vi "Channel Mng Update Test Cases.vi"() -> (0 "error out":errorcluster, 2 "status":string, 3 "pass":bool)   [LabVIEW 2021]
uses:
  <vilib>/CIF Foundation/CIF Channels Core/CIF_NIChn/Double/CIF_NIChn_Double.lvclass
  C:/Program Files/National Instruments/LabVIEW 2021/vi.lib/CIF Foundation/CIF Channels Core/CIFChannels/CIFChannels.lvclass
  <vilib>/CIF Foundation/CIF Channels Core/CIFChannels/Typedef/Direction.ctl
  OOB/OOB_Rx/CIFCoreOOB_Rx.lvclass/CIFCoreOOB_Rx.ctl
  <vilib>/CIF Foundation/CIF Out of Band Commands/CIFOutOfBand.lvclass/CIFOutOfBand.ctl
  <vilib>/CIF Foundation/CIF Channels Core/CIFChannels/CIFChannels.lvclass
  <vilib>/CIF Foundation/CIF Channels Core/CIFChannels/CIFChannels.lvclass/CIFChannels.ctl
  Channels/CIFChannelMng/CIFChannelMng.lvclass/CIFChannelMng.ctl
  OOB/OOB_Rx/Private/Command Settings.vi
  <vilib>/CIF Foundation/CIF Out of Band Commands/Accessors/Write Local OOB Data.vi
  <vilib>/CIF Foundation/CIF Channels Core/ChannelCommon/Utilities/Add Error.vi
  <vilib>/CIF Foundation/CIF Channels Core/CIFChannels/Accessors/Read Name.vi
  <vilib>/CIF Foundation/CIF Channels Core/CIFChannels/Accessors/Read Custom Config Data.vi
  <vilib>/CIF Foundation/CIF Channels Core/CIFChannels/Accessors/Read Type.vi
  <vilib>/CIF Foundation/CIF Channels Core/CIFChannels/Accessors/Read Multi-Writer.vi
  <vilib>/CIF Foundation/CIF Channels Core/CIFChannels/Accessors/Read Direction.vi
  <vilib>/CIF Foundation/CIF Channels Core/CIFChannels/Accessors/Read Channel State.vi
  Channels/CIFChannelMng/Utilities/Get Channel Index by Name.vi
  Channels/CIFChannelMng/Utilities/Remove Channel by Index.vi
  <vilib>/CIF Foundation/CIF Channels Core/CIFChannels/Accessors/Read Tag Forced.vi
  <vilib>/CIF Foundation/CIF Utilities/Errors/Append Error Location.vi
  <vilib>/CIF Foundation/CIF Channels Core/CIFChannels/Accessors/Write Channel State.vi
  OOB/OOB_Rx/CIFCoreOOB_Rx.lvclass
  C:/Program Files/National Instruments/LabVIEW 2021/vi.lib/CIF Foundation/CIF Out of Band Commands/CIFOutOfBand.lvclass
  <vilib>/CIF Foundation/CIF Out of Band Commands/Init OOB.vi
  <vilib>/CIF Foundation/CIF Channels Core/CIFChannels/Core/Set Force.vi
  OOB/OOB_Rx/Typedef/FIFO Publisher.ctl
  <vilib>/CIF Foundation/CIF Channels Core/ChannelCommon/typedef/New FIFO Instance Configuration.ctl
  OOB/OOB_Rx/Typedef/Channel Connection Data.ctl
  Channels/CIFChannelMng/CIFChannelMng.lvclass
  <vilib>/CIF Foundation/CIF Channels Core/CIF_NIChn/FIFO_U8_Multi/CIF_Fifo_U8_Multi.lvclass
  <vilib>/CIF Foundation/CIF Channels Core/ChannelCommon/ChannelCommon.lvlib
  <vilib>/CIF Foundation/CIF Out of Band Commands/CIFOutOfBand.lvclass
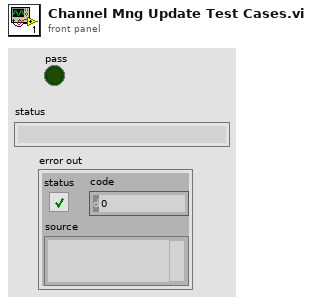
[diagram p1: front panel]
types:
  T1 = typedef "CIFChannels.lvclass/Direction.ctl" = enum16{"Publisher", "Subscriber"}
  T2 = typedef "CIFCoreOOB_Rx.lvclass/Channel Connection Data.ctl" = cluster{"Publisher Name":string, "Subscriber Name":string, "Connection Data":u8[]}
  T3 = typedef "CIFCoreOOB_Rx.lvclass/FIFO Publisher.ctl" = cluster{"Publisher Name":string, "New FIFO Instance Config":T4}
  T4 = typedef "ChannelCommon.lvlib/New FIFO Instance Configuration.ctl" = cluster{"Primary":bool, "Backpressure":bool, "Message/FIFO Override":u32}
  T5 = typedef "ChnMngOOB_Tx.lvclass/FIFO Publisher Return.ctl" = cluster{"FIFO Pub Name":string, "error":errorcluster, "Added":bool}
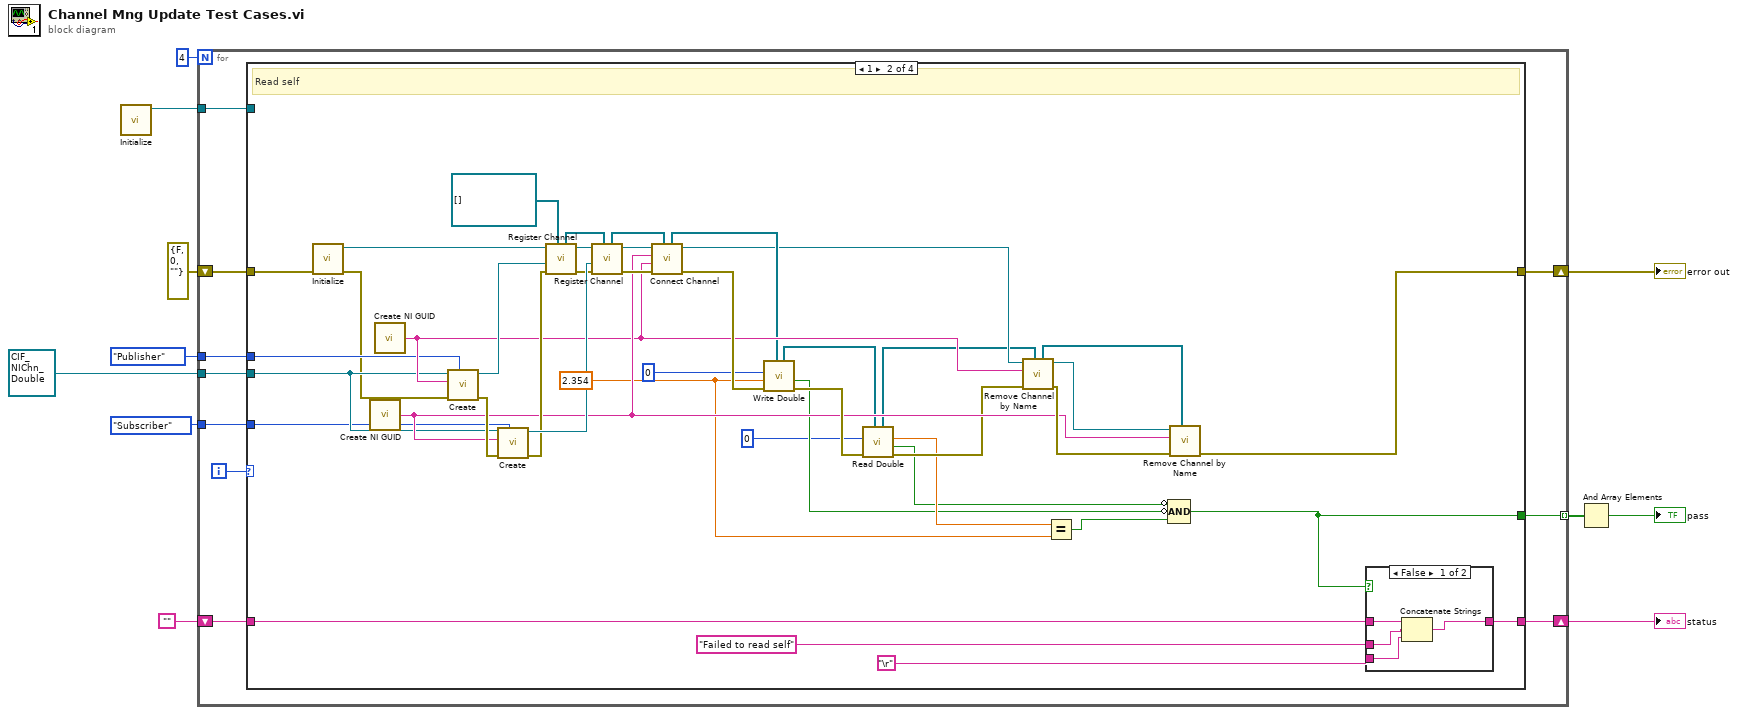
[diagram p0: block diagram]
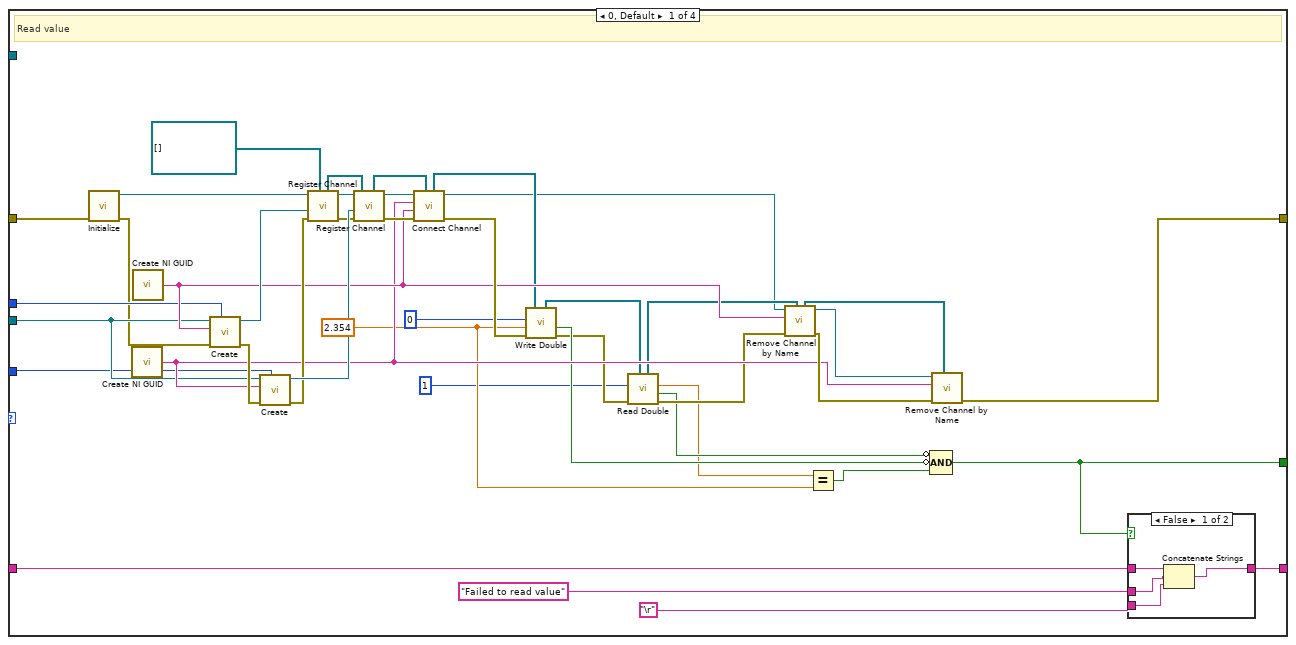
[diagram p2: hidden frame]
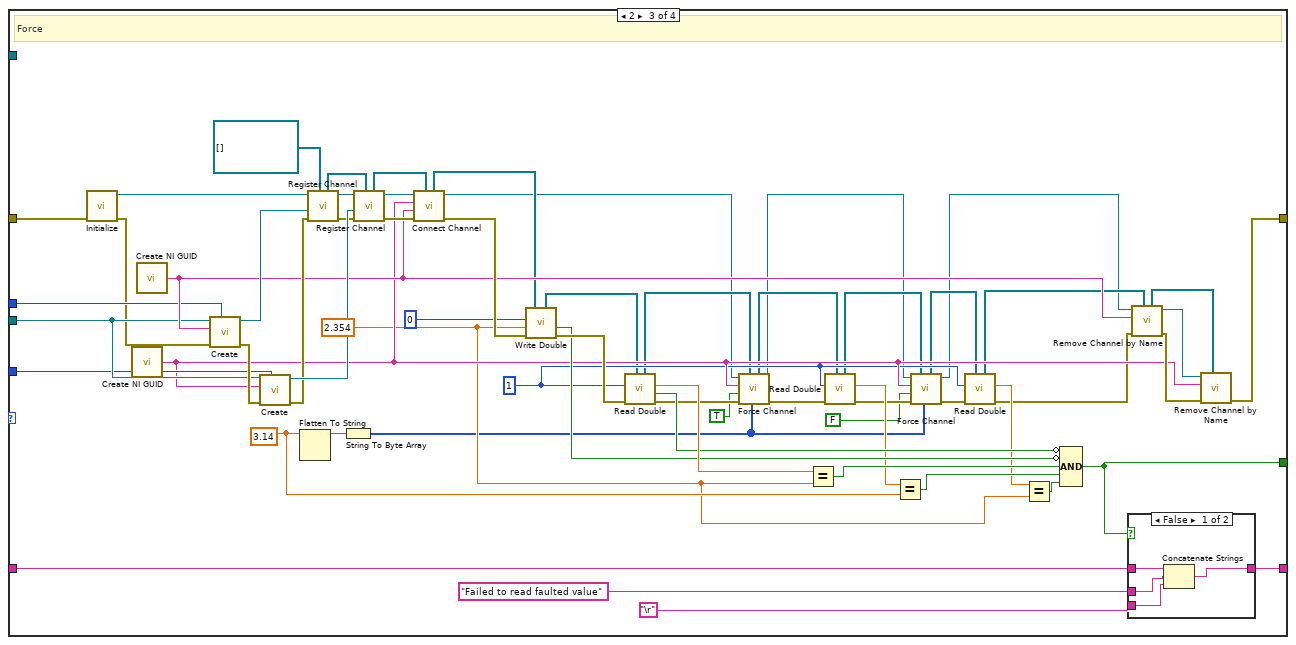
[diagram p5: hidden frame]
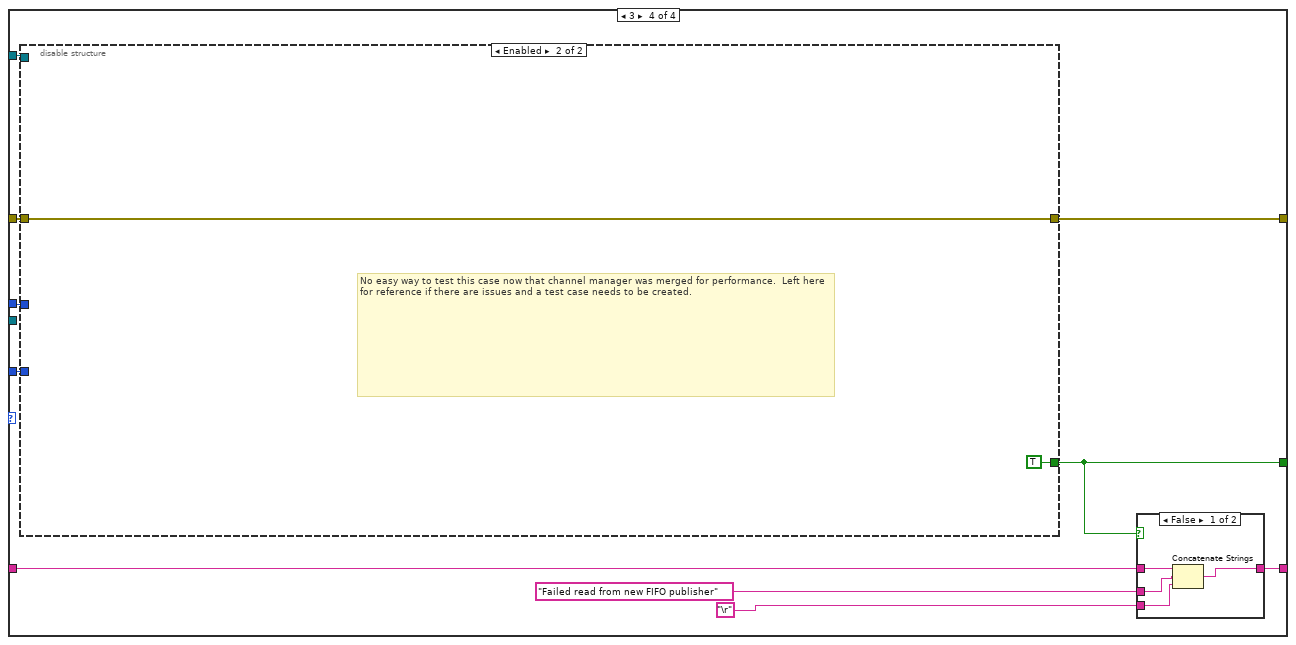
[diagram p7: hidden frame]
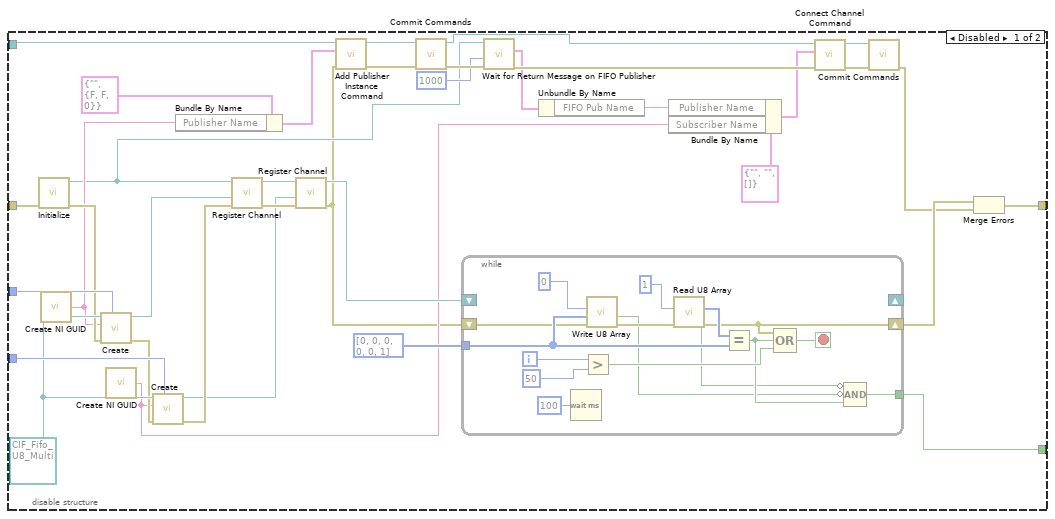
[diagram p8: hidden frame]
diagram:
  n1 = call "Initialize.vi"() -> ("CoreOOB_Rx out"=w1:refnum<class "CIFCoreOOB_Rx.lvclass">)  [unwired: 10 in, 1 out]
  n2 = for {
    N: 4 -> [_]
    tunnel: [w21] -> w11 mode=indexing
    shift-right: [w19] -> w6
    shift-left: errorcluster {"status"=FALSE, "code"=0, "source"=""} ("error out") -> [w20]
    shift-right: [w16] -> w7
    shift-left: "" -> [w17]
    tunnel: refnum<class "CIF_NIChn_Double.lvclass"> refnum ("CIF_NIChn_Double.lvclass") -> [w15]
    tunnel: Direction."Subscriber" ("Direction") -> [w14]
    tunnel: Direction."Publisher" ("Direction") -> [w13]
    tunnel: w1 -> [w12]
    i -> [w18]
    n3 = case shown="1" w18 {
      tunnel: [w58 w105 w171 w187] -> w21
      tunnel: w20 -> [w31 w79 w131 w189]
      tunnel: [w45 w92 w158 w183] -> w19
      tunnel: w17 -> [w63 w110 w176 w186]
      tunnel: [w62 w109 w175 w188] -> w16
      tunnel: w15 -> [w41 w84 w153 _]
      tunnel: w14 -> [w40 w83 w152 w190]
      tunnel: w13 -> [w39 w82 w151 w191]
      tunnel: w12 -> [_ _ _ w182]
      frame 0, Default {
        w43 = 2.354
        # "Read value"
        n4 = call "Initialize.vi"("error in (no error)"=w31) -> ("error out"=w30:errorcluster, "CIFChannelMng out"=w32:refnum<class "CIFChannelMng.lvclass">)  [unwired: 9 in]
        n5 = call <vilib>:"Create NI GUID.vi"() -> ("NI GUID"=w44:string)
        n6 = call <vilib>:"Create NI GUID.vi"() -> ("NI GUID"=w48:string)
        n7 = call-dynamic "Create.vi"("Direction"=w39, "error in (no error)"=w30, "Name"=w48, "CIFTag in"=w41) -> ("error out"=w53:errorcluster, "CIFTag out"=w52:refnum<class "CIF_NIChn_Double.lvclass">)  [unwired: 6 in]
        n8 = call-dynamic "Create.vi"("Direction"=w40, "error in (no error)"=w53, "Name"=w44, "CIFTag in"=w41) -> ("error out"=w54:errorcluster, "CIFTag out"=w57:refnum<class "CIF_NIChn_Double.lvclass">)  [unwired: 6 in]
        n9 = call "Register Channel.vi"("Channel Array in"=refnum<class "CIFChannels.lvclass">[] [], "error in (no error)"=w54, "Channel"=w52, "CIFChannelMng in"=w32) -> ("error out"=w51:errorcluster, "CIFChannelMng out"=w50:refnum<class "CIFChannelMng.lvclass">, "Channel Array out"=w23:refnum<class "CIFChannels.lvclass">[])  [unwired: 4 in, 1 out]
        n10 = call "Register Channel.vi"("Channel Array in"=w23, "error in (no error)"=w51, "Channel"=w57, "CIFChannelMng in"=w50) -> ("error out"=w56:errorcluster, "CIFChannelMng out"=w55:refnum<class "CIFChannelMng.lvclass">, "Channel Array out"=w22:refnum<class "CIFChannels.lvclass">[])  [unwired: 4 in, 1 out]
        n11 = call "Connect Channel.vi"("Channel Array in"=w22, "error in (no error)"=w56, "Publisher Name"=w48, "Subscriber Name"=w44, "CIFChannelMng in"=w55) -> ("error out"=w49:errorcluster, "CIFChannelMng out"=w26:refnum<class "CIFChannelMng.lvclass">, "Channel Array out"=w29:refnum<class "CIFChannels.lvclass">[])  [unwired: 3 in, 1 out]
        n12 = call "Write Double.vi"("Channel Array in"=w29, "error in (no error)"=w49, "Data"=w43, "Channel Index"=0) -> ("error out"=w37:errorcluster, "timed out?"=w42:bool, "Channel Array out"=w28:refnum<class "CIFChannels.lvclass">[])  [unwired: 5 in]
        n13 = call "Read Double.vi"("Channel Array in"=w28, "error in (no error)"=w37, "Channel Index"=1 ("Index")) -> ("error out"=w38:errorcluster, "timed out?"=w35:bool, "Data"=w34:dbl, "Channel Array out"=w27:refnum<class "CIFChannels.lvclass">[])  [unwired: 5 in]
        n14 = call "Remove Channel by Name.vi"("Channel Array in"=w27, "error in (no error)"=w38, "Channel Name"=w48, "CIFChannelMng in"=w26) -> ("error out"=w47:errorcluster, "CIFChannelMng out"=w46:refnum<class "CIFChannelMng.lvclass">, "Channel Array out"=w25:refnum<class "CIFChannels.lvclass">[])  [unwired: 4 in, 1 out]
        n15 = Equal?(x=w34, y=w43) -> (x = y?=w59:bool)
        n16 = Compound Arithmetic op=AND(invert w35, invert w42, w59) -> (w58:bool)
        n17 = call "Remove Channel by Name.vi"("Channel Array in"=w25, "error in (no error)"=w47, "Channel Name"=w44, "CIFChannelMng in"=w46) -> ("error out"=w45:errorcluster)  [unwired: 4 in, 3 out]
        n18 = case shown="False" w58 {
          tunnel: w63 -> [w67 w68]
          tunnel: [w64 w68] -> w62
          tunnel: "Failed to read value" -> [w66 _]
          tunnel: "\r" -> [w65 _]
          frame False {
            n19 = Concatenate Strings(w67, w66, w65) -> (w64:string)
          }
          frame True {
          }
        }
      }
      frame 1 {
        w88 = 2.354
        # "Read self"
        n20 = call "Initialize.vi"("error in (no error)"=w79) -> ("error out"=w77:errorcluster, "CIFChannelMng out"=w78:refnum<class "CIFChannelMng.lvclass">)  [unwired: 9 in]
        n21 = call <vilib>:"Create NI GUID.vi"() -> ("NI GUID"=w91:string)
        n22 = call <vilib>:"Create NI GUID.vi"() -> ("NI GUID"=w85:string)
        n23 = call-dynamic "Create.vi"("Direction"=w82, "error in (no error)"=w77, "Name"=w85, "CIFTag in"=w84) -> ("error out"=w100:errorcluster, "CIFTag out"=w99:refnum<class "CIF_NIChn_Double.lvclass">)  [unwired: 6 in]
        n24 = call-dynamic "Create.vi"("Direction"=w83, "error in (no error)"=w100, "Name"=w91, "CIFTag in"=w84) -> ("error out"=w101:errorcluster, "CIFTag out"=w104:refnum<class "CIF_NIChn_Double.lvclass">)  [unwired: 6 in]
        n25 = call "Register Channel.vi"("Channel Array in"=refnum<class "CIFChannels.lvclass">[] [], "error in (no error)"=w101, "Channel"=w99, "CIFChannelMng in"=w78) -> ("error out"=w98:errorcluster, "CIFChannelMng out"=w97:refnum<class "CIFChannelMng.lvclass">, "Channel Array out"=w76:refnum<class "CIFChannels.lvclass">[])  [unwired: 4 in, 1 out]
        n26 = call "Register Channel.vi"("Channel Array in"=w76, "error in (no error)"=w98, "Channel"=w104, "CIFChannelMng in"=w97) -> ("error out"=w103:errorcluster, "CIFChannelMng out"=w102:refnum<class "CIFChannelMng.lvclass">, "Channel Array out"=w75:refnum<class "CIFChannels.lvclass">[])  [unwired: 4 in, 1 out]
        n27 = call "Connect Channel.vi"("Channel Array in"=w75, "error in (no error)"=w103, "Publisher Name"=w85, "Subscriber Name"=w91, "CIFChannelMng in"=w102) -> ("error out"=w96:errorcluster, "CIFChannelMng out"=w71:refnum<class "CIFChannelMng.lvclass">, "Channel Array out"=w73:refnum<class "CIFChannels.lvclass">[])  [unwired: 3 in, 1 out]
        n28 = call "Write Double.vi"("Channel Array in"=w73, "error in (no error)"=w96, "Data"=w88, "Channel Index"=0) -> ("error out"=w95:errorcluster, "timed out?"=w86:bool, "Channel Array out"=w70:refnum<class "CIFChannels.lvclass">[])  [unwired: 5 in]
        n29 = call "Read Double.vi"("Channel Array in"=w70, "error in (no error)"=w95, "Channel Index"=0) -> ("error out"=w90:errorcluster, "timed out?"=w87:bool, "Data"=w89:dbl, "Channel Array out"=w69:refnum<class "CIFChannels.lvclass">[])  [unwired: 5 in]
        n30 = call "Remove Channel by Name.vi"("Channel Array in"=w69, "error in (no error)"=w90, "Channel Name"=w85, "CIFChannelMng in"=w71) -> ("error out"=w94:errorcluster, "CIFChannelMng out"=w93:refnum<class "CIFChannelMng.lvclass">, "Channel Array out"=w72:refnum<class "CIFChannels.lvclass">[])  [unwired: 4 in, 1 out]
        n31 = Equal?(x=w89, y=w88) -> (x = y?=w106:bool)
        n32 = Compound Arithmetic op=AND(invert w87, invert w86, w106) -> (w105:bool)
        n33 = call "Remove Channel by Name.vi"("Channel Array in"=w72, "error in (no error)"=w94, "Channel Name"=w91, "CIFChannelMng in"=w93) -> ("error out"=w92:errorcluster)  [unwired: 4 in, 3 out]
        n34 = case shown="False" w105 {
          tunnel: w110 -> [w114 w115]
          tunnel: [w111 w115] -> w109
          tunnel: "Failed to read self" -> [w113 _]
          tunnel: "\r" -> [w112 _]
          frame False {
            n35 = Concatenate Strings(w114, w113, w112) -> (w111:string)
          }
          frame True {
          }
        }
      }
      frame 2 {
        w143 = 3.14
        w138 = 1 ("Channel Index")
        w135 = 2.354
        # "Force"
        n36 = call "Initialize.vi"("error in (no error)"=w131) -> ("error out"=w130:errorcluster, "CIFChannelMng out"=w132:refnum<class "CIFChannelMng.lvclass">)  [unwired: 9 in]
        n37 = call <vilib>:"Create NI GUID.vi"() -> ("NI GUID"=w140:string)
        n38 = call <vilib>:"Create NI GUID.vi"() -> ("NI GUID"=w154:string)
        n39 = call-dynamic "Create.vi"("Direction"=w151, "error in (no error)"=w130, "Name"=w154, "CIFTag in"=w153) -> ("error out"=w166:errorcluster, "CIFTag out"=w165:refnum<class "CIF_NIChn_Double.lvclass">)  [unwired: 6 in]
        n40 = call-dynamic "Create.vi"("Direction"=w152, "error in (no error)"=w166, "Name"=w140, "CIFTag in"=w153) -> ("error out"=w167:errorcluster, "CIFTag out"=w170:refnum<class "CIF_NIChn_Double.lvclass">)  [unwired: 6 in]
        n41 = Flatten To String(anything=w143) -> (data string=w147:string)  [unwired: 3 in, 2 out]
        n42 = call "Register Channel.vi"("Channel Array in"=refnum<class "CIFChannels.lvclass">[] [], "error in (no error)"=w167, "Channel"=w165, "CIFChannelMng in"=w132) -> ("error out"=w164:errorcluster, "CIFChannelMng out"=w163:refnum<class "CIFChannelMng.lvclass">, "Channel Array out"=w128:refnum<class "CIFChannels.lvclass">[])  [unwired: 4 in, 1 out]
        n43 = String To Byte Array(string=w147) -> (unsigned byte array=w133:u8[])
        n44 = call "Register Channel.vi"("Channel Array in"=w128, "error in (no error)"=w164, "Channel"=w170, "CIFChannelMng in"=w163) -> ("error out"=w169:errorcluster, "CIFChannelMng out"=w168:refnum<class "CIFChannelMng.lvclass">, "Channel Array out"=w127:refnum<class "CIFChannels.lvclass">[])  [unwired: 4 in, 1 out]
        n45 = call "Connect Channel.vi"("Channel Array in"=w127, "error in (no error)"=w169, "Publisher Name"=w154, "Subscriber Name"=w140, "CIFChannelMng in"=w168) -> ("error out"=w162:errorcluster, "CIFChannelMng out"=w118:refnum<class "CIFChannelMng.lvclass">, "Channel Array out"=w126:refnum<class "CIFChannels.lvclass">[])  [unwired: 3 in, 1 out]
        n46 = call "Write Double.vi"("Channel Array in"=w126, "error in (no error)"=w162, "Data"=w135, "Channel Index"=0) -> ("error out"=w161:errorcluster, "timed out?"=w155:bool, "Channel Array out"=w125:refnum<class "CIFChannels.lvclass">[])  [unwired: 5 in]
        n47 = call "Read Double.vi"("Channel Array in"=w125, "error in (no error)"=w161, "Channel Index"=w138) -> ("error out"=w149:errorcluster, "timed out?"=w156:bool, "Data"=w157:dbl, "Channel Array out"=w124:refnum<class "CIFChannels.lvclass">[])  [unwired: 5 in]
        n48 = call "Force Channel.vi"("Force Data"=w133, "Channel Array in"=w124, "error in (no error)"=w149, "Force Active"=TRUE ("Fault Active"), "Channel Name"=w140, "CIFChannelMng in"=w118) -> ("error out"=w146:errorcluster, "CIFChannelMng out"=w117:refnum<class "CIFChannelMng.lvclass">, "Channel Array out"=w123:refnum<class "CIFChannels.lvclass">[])  [unwired: 2 in, 1 out]
        n49 = Equal?(x=w157, y=w135) -> (x = y?=w172:bool)
        n50 = call "Read Double.vi"("Channel Array in"=w123, "error in (no error)"=w146, "Channel Index"=w138) -> ("error out"=w142:errorcluster, "Data"=w144:dbl, "Channel Array out"=w122:refnum<class "CIFChannels.lvclass">[])  [unwired: 5 in, 1 out]
        n51 = Equal?(x=w144, y=w143) -> (x = y?=w145:bool)
        n52 = call "Force Channel.vi"("Force Data"=w133, "Channel Array in"=w122, "error in (no error)"=w142, "Force Active"=FALSE ("Fault Active"), "Channel Name"=w140, "CIFChannelMng in"=w117) -> ("error out"=w141:errorcluster, "CIFChannelMng out"=w116:refnum<class "CIFChannelMng.lvclass">, "Channel Array out"=w121:refnum<class "CIFChannels.lvclass">[])  [unwired: 2 in, 1 out]
        n53 = call "Read Double.vi"("Channel Array in"=w121, "error in (no error)"=w141, "Channel Index"=w138) -> ("error out"=w134:errorcluster, "Data"=w136:dbl, "Channel Array out"=w120:refnum<class "CIFChannels.lvclass">[])  [unwired: 5 in, 1 out]
        n54 = Equal?(x=w136, y=w135) -> (x = y?=w137:bool)
        n55 = Compound Arithmetic op=AND(invert w156, invert w155, w172, w145, w137) -> (w171:bool)
        n56 = case shown="False" w171 {
          tunnel: w176 -> [w180 w181]
          tunnel: [w177 w181] -> w175
          tunnel: "Failed to read faulted value" -> [w179 _]
          tunnel: "\r" -> [w178 _]
          frame False {
            n57 = Concatenate Strings(w180, w179, w178) -> (w177:string)
          }
          frame True {
          }
        }
        n58 = call "Remove Channel by Name.vi"("Channel Array in"=w120, "error in (no error)"=w134, "Channel Name"=w154, "CIFChannelMng in"=w116) -> ("error out"=w160:errorcluster, "CIFChannelMng out"=w159:refnum<class "CIFChannelMng.lvclass">, "Channel Array out"=w119:refnum<class "CIFChannels.lvclass">[])  [unwired: 4 in, 1 out]
        n59 = call "Remove Channel by Name.vi"("Channel Array in"=w119, "error in (no error)"=w160, "Channel Name"=w140, "CIFChannelMng in"=w159) -> ("error out"=w158:errorcluster)  [unwired: 4 in, 3 out]
      }
      frame 3 {
        n60 = disable-structure shown="Enabled" {
          disable-tunnel: w191 -> [w227 _]
          disable-tunnel: w190 -> [w226 _]
          disable-tunnel: w189 -> [w223 w245]
          disable-tunnel: [w211 TRUE] -> w187
          disable-tunnel: [w210 w245] -> w183
          disable-tunnel: w182 -> [w204 _]
          frame Disabled {
            w225 = refnum<class "CIF_Fifo_U8_Multi.lvclass"> refnum ("CIF_Fifo_U8 in")
            n61 = call "Initialize.vi"("error in (no error)"=w223) -> ("error out"=w222:errorcluster, "CIFChannelMng out"=w203:refnum<class "CIFChannelMng.lvclass">)  [unwired: 9 in]
            n62 = call <vilib>:"Create NI GUID.vi"() -> ("NI GUID"=w214:string)
            n63 = call-dynamic "Create.vi"("Direction"=w227, "error in (no error)"=w222, "Name"=w214, "CIF_Fifo_U8 in"=w225) -> ("error out"=w224:errorcluster, "CIF_Fifo_U8 out"=w221:refnum<class "CIF_Fifo_U8_Multi.lvclass">)  [unwired: 6 in]
            n64 = call <vilib>:"Create NI GUID.vi"() -> ("NI GUID"=w212:string)
            n65 = call-dynamic "Create.vi"("Direction"=w226, "error in (no error)"=w224, "Name"=w212, "CIF_Fifo_U8 in"=w225) -> ("error out"=w220:errorcluster, "CIF_Fifo_U8 out"=w217:refnum<class "CIF_Fifo_U8_Multi.lvclass">)  [unwired: 6 in]
            n66 = Bundle By Name(cluster=T3 {"Publisher Name"="", "New FIFO Instance Config"={"Primary"=FALSE, "Backpressure"=FALSE, "Message/FIFO Override"=0}} ("New Publisher"), "Publisher Name"=w214) -> (w202:T3)
            n67 = call "Register Channel.vi"("error in (no error)"=w220, "Channel"=w221, "CIFChannelMng in"=w203) -> ("error out"=w218:errorcluster, "CIFChannelMng out"=w219:refnum<class "CIFChannelMng.lvclass">)  [unwired: 5 in, 2 out]
            n68 = call "Register Channel.vi"("error in (no error)"=w218, "Channel"=w217, "CIFChannelMng in"=w219) -> ("error out"=w200:errorcluster, "CIFChannelMng out"=w216:refnum<class "CIFChannelMng.lvclass">)  [unwired: 5 in, 2 out]
            n69 = call "Add Publisher Instance Command.vi"("error in"=w200, "New Publisher"=w202, "CoreOOB_Rx in"=w204) -> ("error out"=w207:errorcluster, "CoreOOB_Rx out"=w208:refnum<class "CIFCoreOOB_Rx.lvclass">)  [unwired: 7 in]
            n70 = call <vilib>:"Commit Commands.vi"("error in"=w207, "OOB in"=w208) -> ("error out"=w206:errorcluster, "OOB out"=w197:refnum<class "CIFCoreOOB_Rx.lvclass">)  [unwired: 8 in]
            n71 = while {
              tunnel: u8[] [0, 0, 0, 0, 0, 1] ("Data in") -> [w240]
              shift-right: _ -> [_]
              shift-left: w216 -> [_]
              shift-right: [w235] -> w209
              shift-left: w200 -> [w228]
              tunnel: [w229] -> w211
              i -> [w237]
              stop <- w233 stop-if-true
              n72 = Wait (ms)(milliseconds to wait=u32 100) -> ()  [unwired: 1 out]
              n73 = Greater?(x=w237, y=50) -> (0:w234:bool)
              n74 = call "Write U8 Array.vi"("error in (no error)"=w228, "Data in"=w240, "Channel Index"=0) -> ("error out"=w242:errorcluster, "timed out?"=w230:bool)  [unwired: 6 in, 1 out]
              n75 = call "Read U8 Array.vi"("error in (no error)"=w242, "Channel Index"=1) -> ("error out"=w235:errorcluster, "timed out?"=w231:bool, "Data"=w241:u8[])  [unwired: 5 in, 2 out]
              n76 = Equal?(x=w241, y=w240) -> (x = y?=w232:bool)
              n77 = Compound Arithmetic op=OR(w235, w232, w234) -> (w233:bool)
              n78 = Compound Arithmetic op=AND(invert w231, invert w230, w232) -> (w229:bool)
            }
            n79 = call "Wait for Return Message on FIFO Publisher.vi"("error in (no error)"=w206, "Timeout (ms)"=u32 1000, "CIFChannelMng in"=w203) -> ("error out"=w196:errorcluster, "FIFO Publisher"=w192:T5)  [unwired: 5 in, 2 out]
            n80 = Unbundle By Name(w192) -> ("FIFO Pub Name"=w213:string)
            n81 = Bundle By Name(cluster=T2 {"Publisher Name"="", "Subscriber Name"="", "Connection Data"=[]} ("Channel Connection Data"), "Publisher Name"=w213, "Subscriber Name"=w212) -> (w195:T2)
            n82 = call "Connect Channel Command.vi"("error in"=w196, "Channel Connection Data"=w195, "CoreOOB_Rx in"=w197) -> ("error out"=w198:errorcluster, "CoreOOB_Rx out"=w199:refnum<class "CIFCoreOOB_Rx.lvclass">)  [unwired: 7 in]
            n83 = call <vilib>:"Commit Commands.vi"("error in"=w198, "OOB in"=w199) -> ("error out"=w193:errorcluster)  [unwired: 8 in, 1 out]
            n84 = Merge Errors(w209, w193) -> (w210:errorcluster)
          }
          frame Enabled {
            # "No easy way to test this case now that channel manager was merged for performance.  Left here for reference if there are issues and a test case needs to be created."
          }
        }
        n85 = case shown="False" w187 {
          tunnel: w186 -> [w249 w250]
          tunnel: [w246 w250] -> w188
          tunnel: "Failed read from new FIFO publisher" -> [w248 _]
          tunnel: "\r" -> [w247 _]
          frame False {
            n86 = Concatenate Strings(w249, w248, w247) -> (w246:string)
          }
          frame True {
          }
        }
      }
    }
  }
  "error out" <- w6
  "status" <- w7
  n87 = And Array Elements(Boolean array=w11) -> (logical AND=→"pass":bool)
